vi "MainT.vi"() -> ()   [LabVIEW 2019]
uses:
  <instrlib>/niDMM/nidmm.llb/niDMM Function.ctl
  <instrlib>/niDMM/nidmm.llb/niDMM Resolution in Digits.ctl
panel:
  out "time between obtaining data (ms)":u32
  in  "Self-Calibrate Multimeter at the beginning?":bool
  in  "Tab Control":T1(tab)
  out "Waveform Chart 2":cluster{dbl, dbl, dbl}(graph)
  in  "VISA resource name":refnum<visa-resource-name>="COM3"
  in  "termination char\n(0xA = '\\n' = LF)":u8=13 format="%.0x"
  in  "Recieve Data":bool
  out "Thermometer":dbl(slide) scale=0.0..100.0
  out "Waveform Chart":T2(graph)
  in  "physical channels":tag="PXI1Slot2/ai2"
  in  "resistance configuration":i32(ring)=2 items=["2-Wire"=2, "3-Wire"=3, "4-Wire"=4]
  in  "valor":i32
  out "Waveform Chart 3":dbl(graph)
  out "Measurement (Volts)":dbl format="%_7p"
  out "Over Range?":bool
  in  "Instrument Descriptor":refnum<k15>="PXI1Slot4"
  in  "Function":T3
  in  "Resolution in Digits":T4=5.5 items=["3 1/2"=3.5, "4 1/2"=4.5, "5 1/2"=5.5, "6 1/2"=6.5, "7 1/2"=7.5]
  in  "Range (Volts)":dbl=10.0 format="%.2p"
  in  "stop program":bool
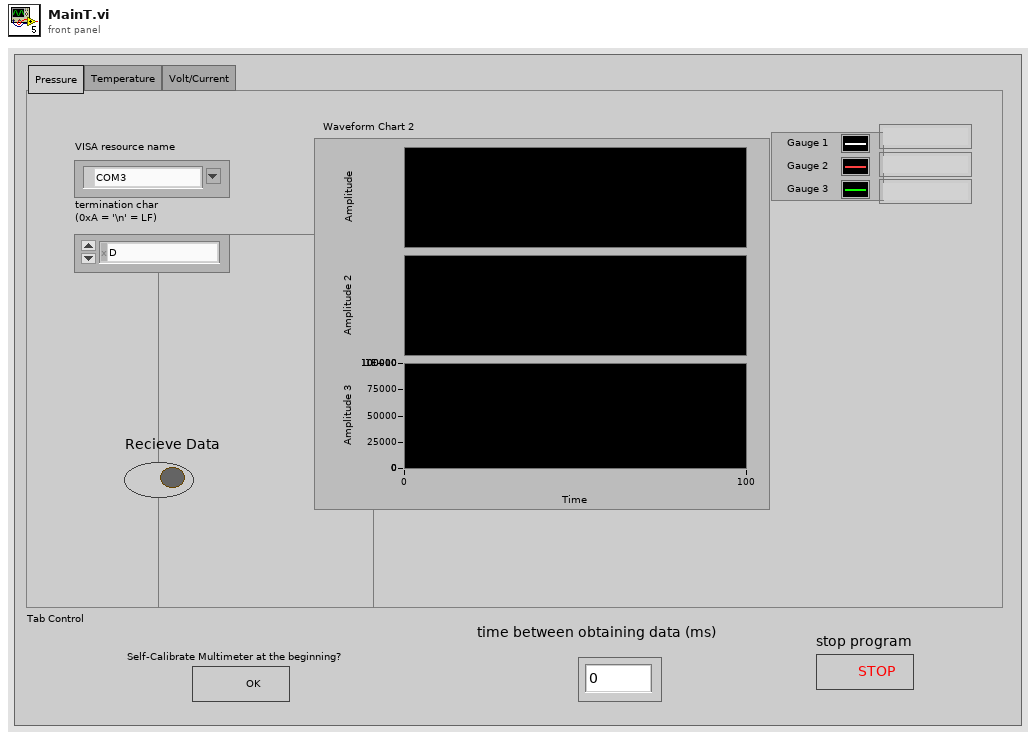
[diagram p1: front panel]
types:
  T1 = enum32{"Pressure", "Temperature", "Volt/Current"}
  T2 = cluster{"data[0]":dbl, "data[1]":dbl, "data[2]":dbl, "data[3]":dbl, "data[4]":dbl, "data[5]":dbl, "data[6]":dbl, "data[7]":dbl, "data[8]":dbl, "data[9]":dbl, "data[10]":dbl, "data[11]":dbl, "data[12]":dbl, "data[13]":dbl, "data[14]":dbl, "data[15]":dbl, "data[16]":dbl, "data[17]":dbl, "data[18]":dbl, "data[19]":dbl}
  T3 = typedef "niDMM Function.ctl" = enum16{"DC Volts", "AC Volts", "DC Current", "AC Current", "2-wire Resistance", "4-wire Resistance", "Diode", "Frequency", "Period", "AC Volts DC Coupled", "Capacitance", "Inductance", "Temperature"}
  T4 = typedef "niDMM Resolution in Digits.ctl" = dbl
  T5 = enum16{"open", "replace", "create", "open or create", "replace or create", "replace or create with confirmation"}
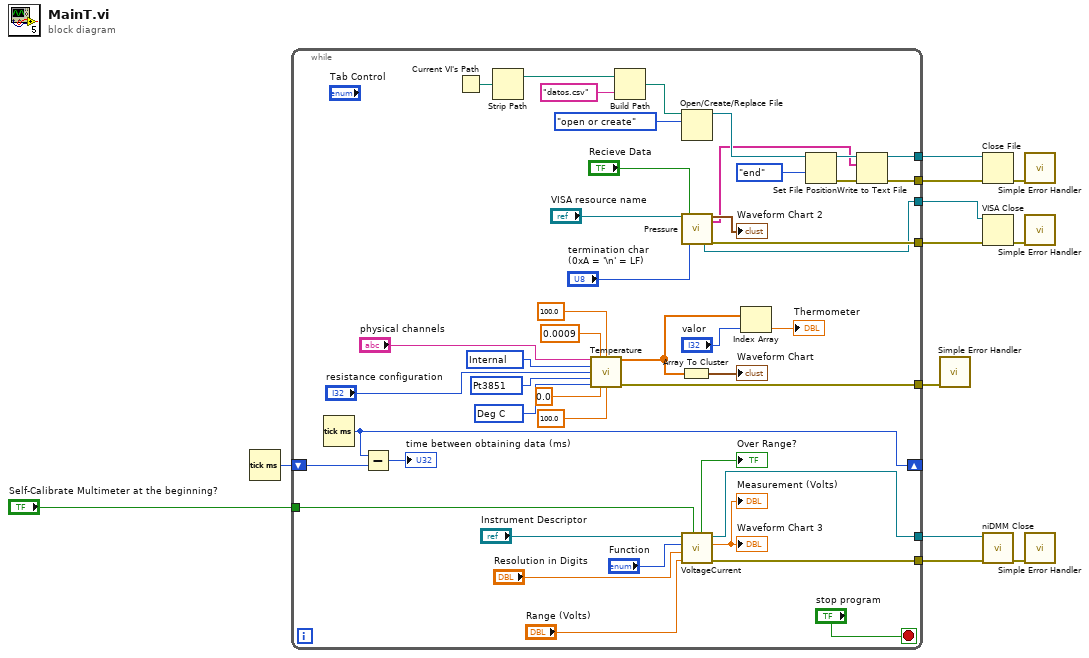
[diagram p0: block diagram]
diagram:
  n1 = Tick Count (ms)() -> (millisecond timer value=w1:u32)
  n2 = while {
    tunnel: [w52] -> w12
    tunnel: [w51] -> w11
    tunnel: [w50] -> w9
    tunnel: [w39] -> w7
    tunnel: [w38] -> w6
    tunnel: "Self-Calibrate Multimeter at the beginning?" -> [w20]
    tunnel: [w18] -> w4
    tunnel: [w17] -> w3
    shift-right: [w14] -> _
    shift-left: w1 -> [w13]
    stop <- "stop program" stop-if-true
    w29 = 10143 items=["Deg C"=10143, "Deg F"=10144, "Kelvins"=10325, "Deg R"=10145, "From Custom Scale"=10065] ("units")
    w30 = 10071 items=["Pt3750"=12481, "Pt3851"=10071, "Pt3911"=12482, "Pt3916"=10069, "Pt3920"=10053, "Pt3928"=12483, "Custom"=10137] ("rtd type")
    w31 = 10200 items=["Internal"=10200, "External"=10167, "None"=10230] ("current excitation source")
    n3 = Tick Count (ms)() -> (millisecond timer value=w14:u32)
    n4 = Subtract(x=w14, y=w13) -> (x-y=→"time between obtaining data (ms)":u32)
    n5 = Current VI's Path() -> (path=w46:path)
    n6 = Strip Path(path=w46) -> (stripped path=w47:path)  [unwired: 1 out]
    n7 = call "Temperature.vi"("physical channels"="physical channels", "current excitation value"=0.0009, "r0"=100.0, "current excitation source"=w31, "resistance configuration"="resistance configuration", "rtd type"=w30, "units"=w29, "minimum value"=0.0, "maximum value"=100.0) -> ("data"=w34:dbl[], "error out"=w50:errorcluster)  [unwired: 4 in, 1 out]
    n8 = Build Path(base path=w47, name or relative path="datos.csv") -> (appended path=w48:path)
    n9 = Array To Cluster(array=w34) -> (cluster=→"Waveform Chart":T2)
    n10 = Open/Create/Replace File(file path (use dialog)=w48, operation (0:open)=T5."open or create") -> (refnum out=w49:refnum<file>)  [unwired: 4 in, 2 out]
    n11 = call "Pressure.vi"("VISA resource name"="VISA resource name", "Recieve Data"="Recieve Data", "termination char\n(0xA = '\\n' = LF)"="termination char\n(0xA = '\\n' = LF)") -> ("VISA resource name out"=w51:refnum<visa-resource-name>, "output cluster"=→"Waveform Chart 2":cluster{dbl, dbl, dbl}, "output array"=w40:string[], "error out"=w52:errorcluster)  [unwired: 10 in, 3 out]
    n12 = call "VoltageCurrent.vi"("Self-Calibrate at the beginning?"=w20, "Range (Volts)"="Range (Volts)", "Resolution in Digits"="Resolution in Digits", "Function"="Function", "Instrument Descriptor"="Instrument Descriptor") -> ("error out"=w17:errorcluster, "Measurement (Volts)"=→"Measurement (Volts)" →"Waveform Chart 3":dbl, "instrument handle out"=w18:refnum<k15>, "Over Range?"=→"Over Range?":bool)  [unwired: 2 in, 1 out]
    n13 = Index Array(array=w34, index="valor") -> (element=→"Thermometer":dbl)
    n14 = Set File Position(refnum=w49, from (0:start)=enum16{"start", "end", "current"}."end") -> (refnum out=w42:refnum<file>, error out=w41:errorcluster)  [unwired: 2 in]
    n15 = Write to Text File(file (use dialog)=w42, text=w40, error in=w41) -> (refnum out=w39:refnum<file>, error out=w38:errorcluster)  [unwired: 1 in, 1 out]
  }
  n16 = call <vilib>:"Simple Error Handler.vi"("error in (no error)"=w9) -> ()  [unwired: 4 in, 5 out]
  n17 = Close File(refnum=w7, error in=w6) -> (error out=w8:errorcluster)  [unwired: 1 out]
  n18 = VISA Close(VISA resource name=w11, error in (no error)=w12) -> (error out=w10:errorcluster)
  n19 = call <instrlib>:"niDMM Close.vi"("error in (no error)"=w3, "instrument handle"=w4) -> ("error out"=w2:errorcluster)  [unwired: 9 in]
  n20 = call <vilib>:"Simple Error Handler.vi"("error in (no error)"=w8) -> ()  [unwired: 1 in, 8 out]
  n21 = call <vilib>:"Simple Error Handler.vi"("error in (no error)"=w10) -> ()  [unwired: 4 in, 5 out]
  n22 = call <vilib>:"Simple Error Handler.vi"("error in (no error)"=w2) -> ()  [unwired: 4 in, 5 out]
